vi "Config Load Sequence.vi"(8 "Sys Error In":errorcluster, 9 "Base Path":path, 10 "Station":string, 11 "Part Type":string) -> (0 "Sys Error Out":errorcluster, 1 "Sequence Name":string, 2 "Item Names":string[][](array[string]), 3 "Seqence Info":T1[](array[typedef]))   [LabVIEW 2018]
uses:
  type defs/Sequence Info.ctl
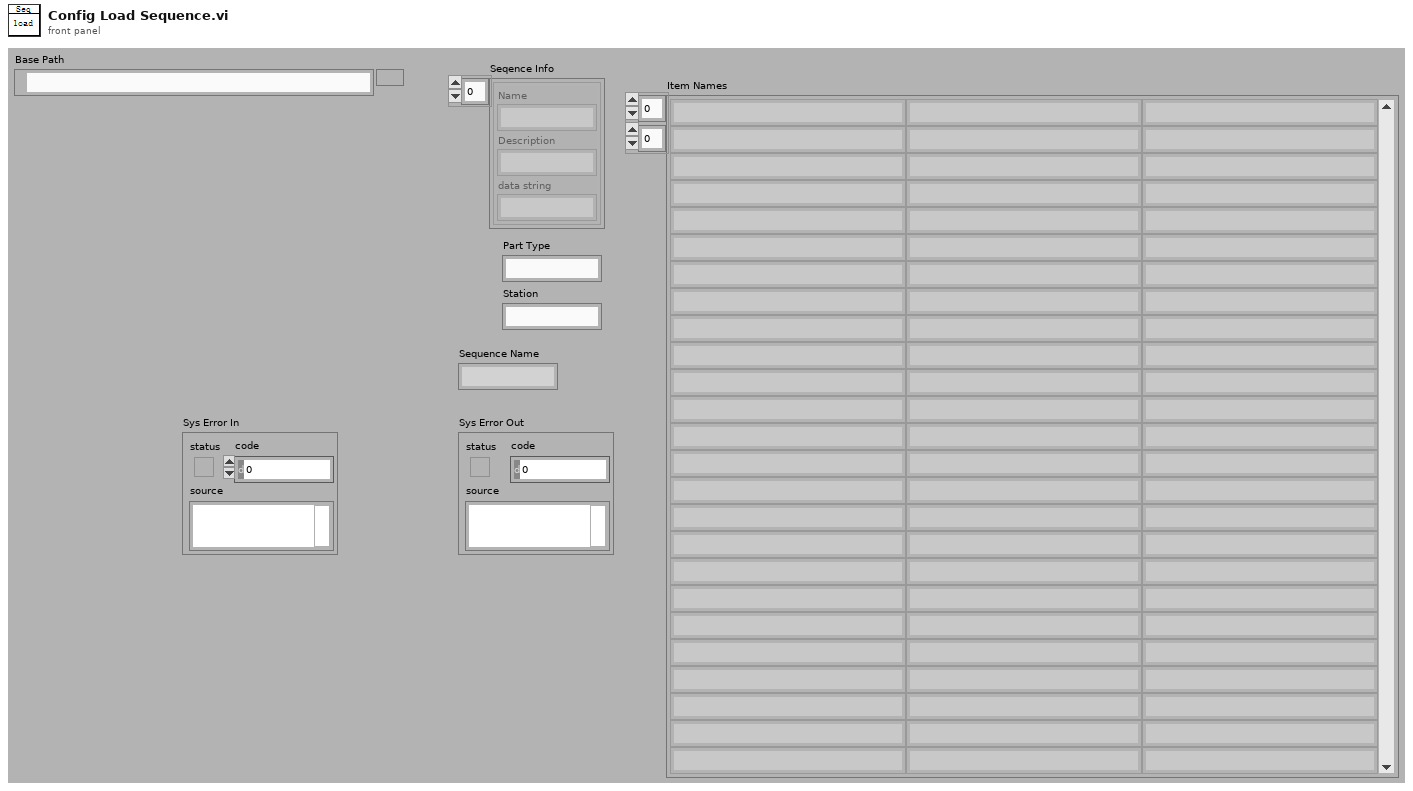
[diagram p1: front panel]
types:
  T1 = typedef "Sequence Info.ctl" = cluster{"Name":string, "Description":string, "data string":string}
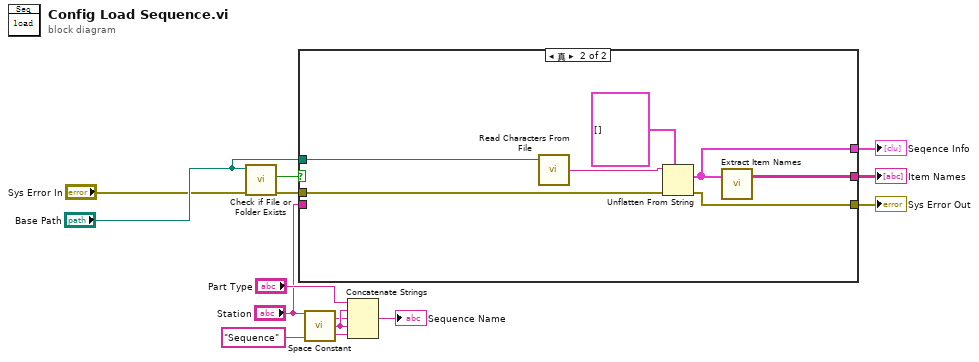
[diagram p0: block diagram]
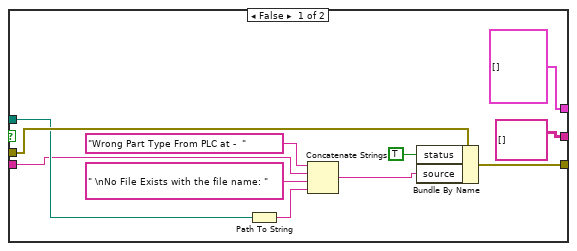
[diagram p2: hidden frame]
diagram:
  n1 = call <vilib>:"Check if File or Folder Exists.vi"("error in (no error)"="Sys Error In", "path"="Base Path") -> ("error out"=w4:errorcluster, "file or folder exists?"=w12:bool)  [unwired: 7 in, 1 out]
  n2 = case shown="真" w12 {
    tunnel: "Base Path" -> [w19 w28]
    tunnel: [T1[] [] ("Seqence Info") w27] -> w11
    tunnel: [string[][] [] ("Item Names") w26] -> w10
    tunnel: w4 -> [w20 w25]
    tunnel: [w18 w24] -> w5
    tunnel: "Station" -> [w13 _]
    frame False {
      n3 = Path To String(path=w19) -> (string=w22:string)
      n4 = Concatenate Strings("Wrong Part Type From PLC at -  " ("string"), w13, " \nNo File Exists with the file name: " ("string"), w22) -> (w21:string)
      n5 = Bundle By Name(cluster=w20, "status"=TRUE, "source"=w21) -> (w18:errorcluster)
    }
    frame True {
      n6 = call <vilib>:"Read Characters From File.vi"("file path (dialog if empty)"=w28) -> ("character string"=w30:string)  [unwired: 5 in, 3 out]
      n7 = Unflatten From String(type=T1[] [] ("Seqence Info"), binary string=w30, error in (no error)=w25) -> (value=w27:T1[], error out=w24:errorcluster)  [unwired: 2 in, 1 out]
      n8 = call "Extract Item Names.vi"("Step Array"=w27) -> ("Item Names"=w26:string[][])  [unwired: 2 in]
    }
  }
  "Seqence Info" <- w11
  "Item Names" <- w10
  "Sys Error Out" <- w5
  n9 = call <vilib>:"Space Constant.vi"() -> ("String"=w6:string)
  n10 = Concatenate Strings("Part Type", w6, "Station", w6, "Sequence" ("string")) -> (→"Sequence Name":string)
